vi "STFT by Increment.vi"(0 "scaled signal [EU]":dbl[](array[numeric]) format="%.2f", 1 "frequency weighting":T4(ring), 5 "sampling frequency [Hz]":dbl=10000.0 format="%.2f", 7 "FFT info":T1={"FFT block size"=1024, "number of FFT"=0, "start index"=0, "increment"=0.0} {"increment" format="%.2f"}, 9 "window":T3 items=["Rectangle"=0, "Hanning"=1, "Hamming"=2, "Blackman-Harris"=3, "Exact Blackman"=4, "Blackman"=5, "Flat Top"=6, "4 Term B-Harris "=7, "7 Term B-Harris"=8, "Low Sidelobe"=9, "Blackman Nuttall"=11, "Triangle"=30, "Bartlett-Hanning"=31, "Bohman"=32, "Parzen"=33, "Welch"=34, "Kaiser"=60, "Dolph-Chebyshev"=61, "Gaussian"=62], 11 "channel info":T2={"sensor sensitivity [mV/EU]"=1000.0, "engineering units"=enum."V", "dB reference [EU]"=1.0, "custom label"="EU", "weighting filter"=enum."Linear", "pregain [dB]"=0.0} {"dB reference [EU]" format="%.1e"; "pregain [dB]" format="%.2f"; "sensor sensitivity [mV/EU]" format="%.2f"}, 12 "dB On (T)":bool=TRUE) -> (4 "power spectrum [EU^2 rms]":dbl[][](array[numeric]) format="%.2f", 6 "unit label":string, 8 "f0 and delta f [Hz]":cluster{"f0":dbl, "delta f":dbl} {"delta f" format="%.2f"; "f0" format="%.2f"}, 15 "weighting conflict":bool)   [LabVIEW 2017]
uses:
  <vilib>/Analysis/4window.llb/windowTd.ctl
  <vilib>/Analysis/NI_AALPro.lvlib
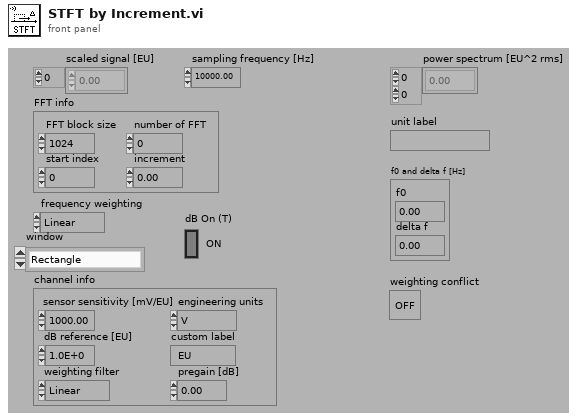
[diagram p1: front panel]
types:
  T1 = cluster{"FFT block size":i32, "number of FFT":i32, "start index":i32, "increment":dbl}
  T2 = cluster{"sensor sensitivity [mV/EU]":dbl, "engineering units":enum16{"custom...", "V", "Pa", "g", "m/s^2", "m/s", "m", "in/s^2", "in/s", "in"}, "dB reference [EU]":dbl, "custom label":string, "weighting filter":enum16{"Linear", "A-weighting", "B-weighting", "C-weighting"}, "pregain [dB]":dbl}
  T3 = typedef "NI_AALPro.lvlib/windowTd.ctl" = u32
  T4 = enum16{"Linear", "A-weighting", "B-weighting", "C-weighting"}
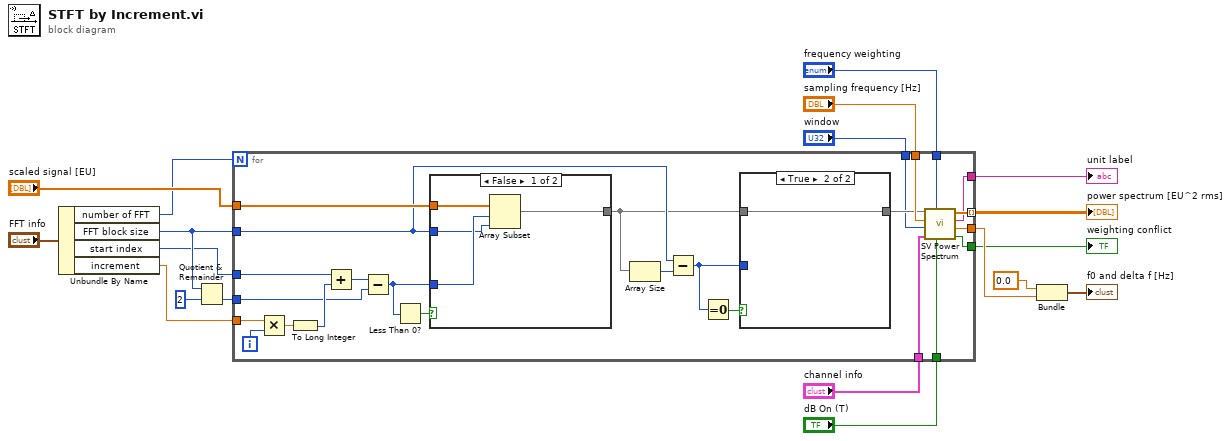
[diagram p0: block diagram]
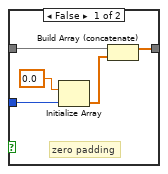
[diagram p2: hidden frame]
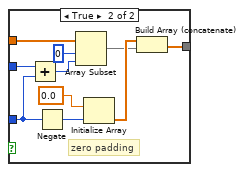
[diagram p3: hidden frame]
diagram:
  n1 = Unbundle By Name("FFT info") -> ("number of FFT"=w3:i32, "FFT block size"=w4:i32, "start index"=w2:i32, "increment"=w1:dbl)
  n2 = Quotient & Remainder(x=w4, y=2) -> (floor(x/y)=w18:i32)  [unwired: 1 out]
  n3 = for {
    N: w3 -> [_]
    tunnel: w2 -> [w44]
    tunnel: w1 -> [w43]
    tunnel: w18 -> [w38]
    tunnel: "scaled signal [EU]" -> [w36]
    tunnel: w4 -> [w35]
    tunnel: "sampling frequency [Hz]" -> [w32]
    tunnel: [w31] -> w17 mode=indexing
    tunnel: [w29] -> w16
    tunnel: "frequency weighting" -> [w25]
    tunnel: "window" -> [w24]
    tunnel: "channel info" -> [w23]
    tunnel: "dB On (T)" -> [w22]
    tunnel: [w21] -> w8
    tunnel: [w20] -> w7
    i -> [w42]
    n4 = Multiply(x=w43, y=w42) -> (x*y=w41:dbl)
    n5 = To Long Integer(number=w41) -> (32bit integer=w40:i32)
    n6 = Add(x=w44, y=w40) -> (x+y=w39:i32)
    n7 = Subtract(x=w39, y=w38) -> (x-y=w37:i32)
    n8 = Less Than 0?(x=w37) -> (x < 0?=w30:bool)
    n9 = case shown="False" w30 {
      tunnel: w37 -> [w53 w60]
      tunnel: w36 -> [w54 w62]
      tunnel: w35 -> [w52 w58]
      tunnel: [w51 w55] -> w34
      frame False {
        n10 = Array Subset(array=w54, index=w53, length=w52) -> (w51:dbl[])
      }
      frame True {
        # "zero padding"
        n11 = Add(x=w58, y=w60) -> (x+y=w59:i32)
        n12 = Negate(x=w60) -> (-x=w64:i32)
        n13 = Array Subset(array=w62, index=0, length=w59) -> (w56:dbl[])
        n14 = Initialize Array(0.0, w64) -> (w57:dbl[])
        n15 = Build Array (concatenate)(w57, w56) -> (w55:dbl[])
      }
    }
    n16 = Array Size(array=w34) -> (size(s)=w28:i32)
    n17 = Subtract(x=w35, y=w28) -> (x-y=w33:i32)
    n18 = Equal To 0?(x=w33) -> (x = 0?=w27:bool)
    n19 = case shown="True" w27 {
      tunnel: [w45 w50] -> w26
      tunnel: w34 -> [w49 w50]
      tunnel: w33 -> [w47 _]
      frame False {
        # "zero padding"
        n20 = Initialize Array(0.0, w47) -> (w46:dbl[])
        n21 = Build Array (concatenate)(w49, w46) -> (w45:dbl[])
      }
      frame True {
      }
    }
    n22 = call <vilib>:"SV Power Spectrum.vi"("dB On (F)"=w22, "frequency weighting"=w25, "channel info"=w23, "window"=w24, "sampling frequency [Hz]"=w32, "scaled signal [EU]"=w26) -> ("weighting conflict"=w20:bool, "df [Hz]"=w29:dbl, "unit label"=w21:string, "power spectrum [EU^2 rms]"=w31:dbl[])  [unwired: 1 in, 1 out]
  }
  "power spectrum [EU^2 rms]" <- w17
  "unit label" <- w8
  "weighting conflict" <- w7
  n23 = Bundle(0.0, "df [Hz]"=w16) -> (→"f0 and delta f [Hz]":cluster{dbl, "df [Hz]":dbl})  [unwired: 1 in]
